vi "Platform Launch.vi"   [LabVIEW 2019, in "Platform.lvlib"]
uses:
  Platform/Platform.lvclass
  C:/Program Files (x86)/National Instruments/LabVIEW 2019/vi.lib/MGI/Panel Manager/Panel Actor/Panel Actor/Panel Actor.lvclass
  <vilib>/MGI/Panel Manager/Panel/Window Position/Reference Position/Ref Display/Ref Display.lvclass
  C:/Program Files (x86)/National Instruments/LabVIEW 2019/vi.lib/MGI/Panel Manager/Panel/Window Position/Window Position.lvclass
  <vilib>/MGI/Panel Manager/Panel Actor/Panel Actor/Launch Root Panel Window.vi
  Platform.lvlib
  <vilib>/MGI/Panel Manager/Panel Actor/Panel Actor/Panel Actor.lvclass
  <vilib>/MGI/Panel Manager/Panel/Panel.lvlib
  <vilib>/MGI/Panel Manager/Panel/Window Position/Reference Position/Vertical Alignment.ctl
  <vilib>/MGI/Panel Manager/Panel/Window Position/Reference Position/Reference Position.lvclass
  <vilib>/MGI/Panel Manager/Panel/Window Position/Reference Position/Horizontal Alignment.ctl
  <vilib>/MGI/Panel Manager/Panel/Window Position/Reference Position/Alignment.ctl
  <vilib>/MGI/Panel Manager/Panel/Window Position/Reference Position/Offset/Absolute Offset/No Offset.vi
  <vilib>/MGI/Panel Manager/Panel/Window Position/Reference Position/Offset/Absolute Offset/Absolute Offset.lvclass
  <vilib>/MGI/Panel Manager/Panel/Window Position/Reference Position/Ref Display/Ref Display.vi
  C:/Program Files (x86)/National Instruments/LabVIEW 2019/vi.lib/MGI/Panel Manager/Panel/Window Position/Reference Position/Offset/Offset.lvclass
  C:/Program Files (x86)/National Instruments/LabVIEW 2019/vi.lib/MGI/Panel Manager/Panel/Window Position/Reference Position/Reference Position.lvclass
  C:/Program Files (x86)/National Instruments/LabVIEW 2019/vi.lib/MGI/Monitored Actor/Monitored Actor/Monitored Actor/Monitored Actor.lvclass
  C:/Program Files (x86)/National Instruments/LabVIEW 2019/vi.lib/ActorFramework/Actor/Actor.lvclass
panel:
  # "Test Launcher"
types:
  T1 = enum32{"Invalid", "Standard", "Closed", "Hidden", "Minimized", "Maximized"}
  T2 = typedef "Panel.lvlib/Reference Position.lvclass/Alignment.ctl" = cluster{"Horizontal":T3, "Vertical":T4}
  T3 = typedef "Panel.lvlib/Reference Position.lvclass/Horizontal Alignment.ctl" = enum16{"Left", "Center", "Right"}
  T4 = typedef "Panel.lvlib/Reference Position.lvclass/Vertical Alignment.ctl" = enum16{"Top", "Center", "Bottom"}
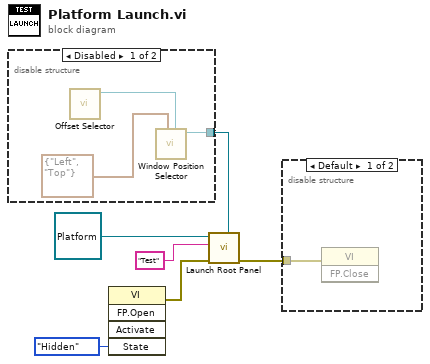
[diagram p0: block diagram]
diagram:
  n1 = disable-structure shown="Disabled" {
    disable-tunnel: [w7 _] -> w3
    frame Disabled {
      n2 = call-poly <vilib>:"Offset Selector.vi"() -> ("Absolute Offset Out"=w9:refnum<class "Absolute Offset.lvclass">)  [unwired: 10 in, 1 out]
      n3 = call-poly <vilib>:"Window Position Selector.vi"("Offset"=w9, "Alignment"=T2 {"Horizontal"=enum."Left", "Vertical"=enum."Top"}) -> ("Ref Display out"=w7:refnum<class "Ref Display.lvclass">)  [unwired: 8 in, 1 out]
    }
    frame Enabled {
    }
  }
  n4 = invoke class="VI" method="FP.Open"("State"=T1."Hidden") -> (error out=w2:errorcluster)  [unwired: 4 in, 4 out]
  n5 = call-poly <vilib>:"Launch Root Panel.vi"("Window Position (Maximize First Call)"=w3, "Error In"=w2, "Title"="Test", "Panel Actor in"=refnum<class "Platform.lvclass"> refnum ("Platform.lvlib:Platform.lvclass")) -> ("Error Out"=w5:errorcluster)  [unwired: 6 in, 1 out]
  n6 = disable-structure shown="Default" {
    disable-tunnel: w5 -> [w10 _]
    frame condition #0 {
      n7 = invoke class="VI" method="FP.Close"(error in=w10) -> ()  [unwired: 2 in, 3 out]
    }
    frame condition #1 (active) {
    }
  }
